vi "unused_new.vi"(8 "error in (no error)":errorcluster, 11 "NotifierStopMechanism in":refnum<class "NotifierStopMechanism.lvclass">) -> (0 "error out":errorcluster, 3 "NotifierStopMechanism out":refnum<class "NotifierStopMechanism.lvclass">)   [LabVIEW 2023]
uses:
  NotifierStopMechanism.lvclass/NotifierStopMechanism.ctl
  NotifierStopMechanism.lvclass
  C:/projects/TLC_Daemon/source/NotifierStopMechanism/NotifierStopMechanism.lvclass
  C:/projects/TLC_Daemon/source/ITaskStopMechanism/ITaskStopMechanism.lvclass
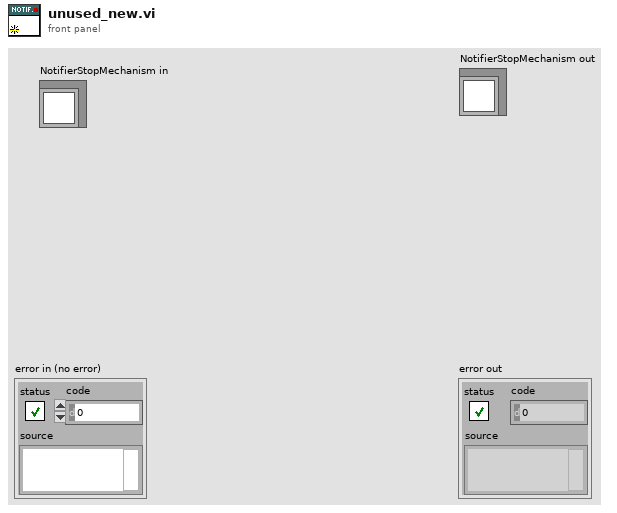
[diagram p1: front panel]
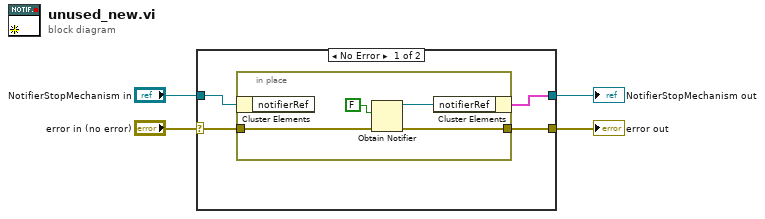
[diagram p0: block diagram]
diagram:
  n1 = case shown="No Error" "error in (no error)" {
    selector: "error in (no error)" -> [w8 w14]
    tunnel: [w7 w14] -> w3
    tunnel: [w5 w13] -> w2
    tunnel: "NotifierStopMechanism in" -> [w6 w13]
    frame No Error {
      n2 = in-place {
        in-place-border: w8 -> [w11]
        in-place-border: [w10] -> w7
        n3 = in-place-cluster #1(w6) -> ()  [unwired: 1 out]
        n4 = Obtain Notifier(notification data type=FALSE, error in (no error)=w11) -> (notifier out=w9:refnum<notifier>, error out=w10:errorcluster)  [unwired: 2 in, 1 out]
        n5 = in-place-cluster #1("notifierRef"=w9) -> (w5:cluster{})
      }
    }
    frame Error {
    }
  }
  "error out" <- w3
  "NotifierStopMechanism out" <- w2
